vi "Abort Request.vi"(8 "error in (no error)":errorcluster, 11 "Requestor":string) -> (0 "error out":errorcluster)   [LabVIEW 2018, in "Test.lvclass"]
uses:
  Test.lvclass
  SSMEventType.ctl
  <vilib>/Utility/error.llb/Error Cluster From Error Code.vi
  <vilib>/ErrorRing/Error Ring.xnode
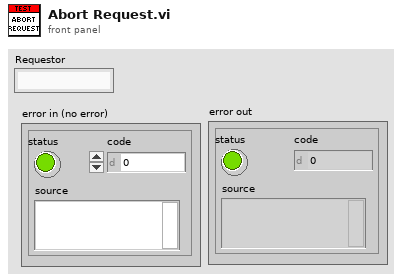
[diagram p1: front panel]
types:
  T1 = typedef "Test.lvclass/SSMRequestEvents.ctl" = cluster{"ShowPanel":refnum<user-event>, "Abort":refnum<user-event>}
  T2 = typedef "Test.lvclass/SSMEventType.ctl" = cluster{"Requester":string, "Data":variant}
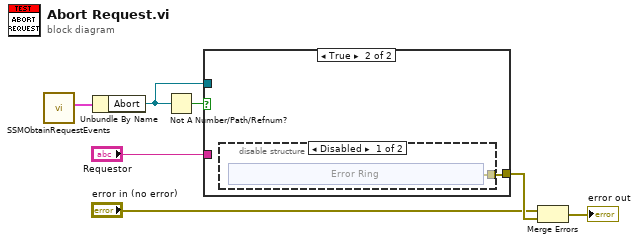
[diagram p0: block diagram]
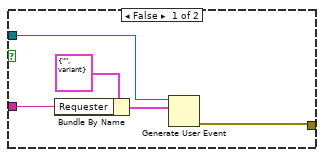
[diagram p2: hidden frame]
diagram:
  n1 = call "SSMObtainRequestEvents.vi"() -> ("SSMRequestEvents"=w1:T1)  [unwired: 10 in, 1 out]
  n2 = Unbundle By Name(w1) -> ("Abort"=w6:refnum<user-event>)
  n3 = Not A Number/Path/Refnum?(number/path/refnum=w6) -> (NaN/Path/Refnum?=w7:bool)
  n4 = case shown="True" w7 {
    tunnel: w6 -> [w11 _]
    tunnel: "Requestor" -> [w8 _]
    tunnel: [w10 w13] -> w3
    frame False {
      n5 = Bundle By Name(cluster=T2 {"Requester"="", "Data"=variant} ("clEventType"), "Requester"=w8) -> (w12:T2)
      n6 = Generate User Event(user event=w11, event data cluster=w12) -> (error out=w10:errorcluster)  [unwired: 2 in, 1 out]
    }
    frame True {
      n7 = disable-structure shown="Disabled" {
        disable-tunnel: [w14 _] -> w13
        frame Disabled {
          n8 = xnode "Error Ring"() -> ("error out"=w14:errorcluster)
        }
        frame Enabled {
        }
      }
    }
  }
  n9 = Merge Errors("error in (no error)", w3) -> (→"error out":errorcluster)
